vi "Execute Value Update Policy.vi"(8 "error in (no error)":errorcluster, 9 "Publish Time":timestamp, 10 "New Topic Value":variant, 11 "ValueChangeSubscription In":refnum<class "ValueChangeSubscription.lvclass">) -> (0 "error out":errorcluster, 3 "ValueChangeSubscription Out":refnum<class "ValueChangeSubscription.lvclass">)   [LabVIEW 2020, in "SubscriptionPolicy.lvlib" / "ValueChangeSubscription.lvclass"]
uses:
  <vilib>/gpm_packages/@cs/mva-core/Source/SubscriptionPolicy/ValueChangeSubscription/ValueChangeSubscription.lvclass
  C:/Program Files/National Instruments/LabVIEW 2020/vi.lib/gpm_packages/@cs/mva-core/Source/IMediator/ISubscriptionPolicy/ISubscriptionPolicy.lvclass
  <vilib>/gpm_packages/@cs/mva-core/Source/SubscriptionPolicy/ValueChangeSubscription/ValueChangeSubscription.lvclass/ValueChangeSubscription.ctl
  <vilib>/gpm_packages/@cs/mva-core/Source/IMediator/ISubscriptionPolicy/ISubscriptionPolicy.lvclass/ISubscriptionPolicy.ctl
  <vilib>/gpm_packages/@cs/transport/Source/ITransport/Transport Data.vi
  <vilib>/gpm_packages/@cs/transport/Source/ITransport/ITransport.lvclass
  <vilib>/gpm_packages/@cs/mva-core/Source/IMediator/ISubscriptionPolicy/ISubscriptionPolicy.lvclass
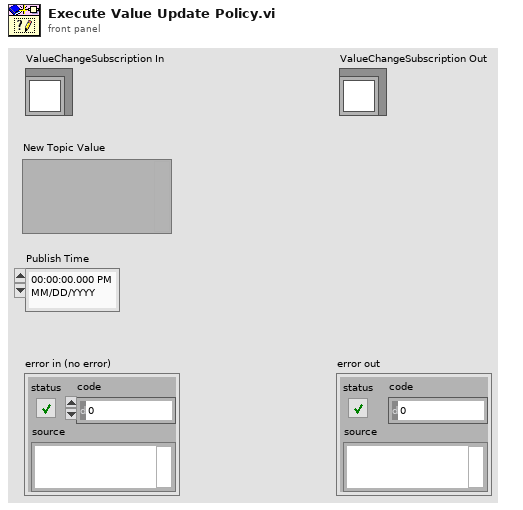
[diagram p1: front panel]
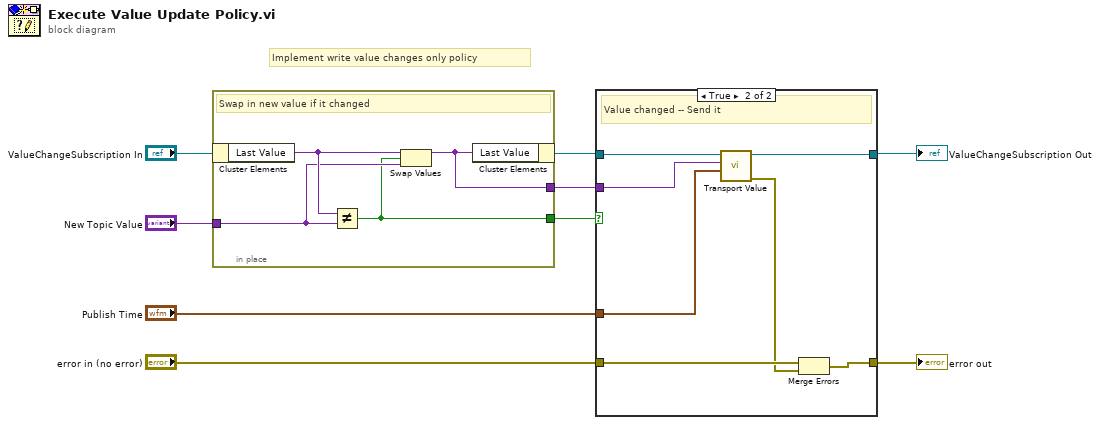
[diagram p0: block diagram]
diagram:
  # "Implement write value changes only policy"
  n1 = in-place {
    in-place-border: "New Topic Value" -> [w12]
    in-place-border: [w11] -> w5
    in-place-border: [w10] -> w1
    # "Swap in new value if it changed"
    n2 = in-place-cluster #1("ValueChangeSubscription In") -> ("Last Value"=w13:variant)
    n3 = Not Equal?(x=w13, y=w12) -> (x != y?=w11:bool)
    n4 = Swap Values(12:w13, 13:w11, 14:w12) -> (1:w10:variant)  [unwired: 1 out]
    n5 = in-place-cluster #1("Last Value"=w10) -> (w2:refnum<class "ValueChangeSubscription.lvclass">)
  }
  n6 = case shown="True" w5 {
    tunnel: "Publish Time" -> [_ w18]
    tunnel: "error in (no error)" -> [w14 w22]
    tunnel: [w14 w21] -> w6
    tunnel: w2 -> [w15 w20]
    tunnel: [w15 w17] -> w4
    tunnel: w1 -> [_ w16]
    frame False {
      # "No value change -- Do nothing"
    }
    frame True {
      # "Value changed -- Send it"
      n7 = call <vilib>:"Transport Value.vi"("Publish Time"=w18, "Value"=w16, "ISubscriptionPolicy in"=w20) -> ("error out"=w19:errorcluster, "ISubscriptionPolicy out"=w17:refnum<class "ValueChangeSubscription.lvclass">)  [unwired: 7 in]
      n8 = Merge Errors(w22, w19) -> (w21:errorcluster)
    }
  }
  "error out" <- w6
  "ValueChangeSubscription Out" <- w4
